vi "read pair information.vi"(8 "error in":errorcluster, 11 "UDP Broadcast Editor Node in":refnum<class "TEC editor node.lvclass">) -> (0 "error out":errorcluster, 2 "pair info":T1, 3 "UDP Broadcast Editor Node out":refnum<class "TEC editor node.lvclass">)   [LabVIEW 2013, in "TEC editor node.lvclass"]
uses:
  TEC editor node.lvclass
  pair information.ctl
  pair type.ctl
  TEC editor node.lvclass/TEC editor node.ctl
  <vilib>/NI/Tag Bus Module Framework/root configuration/TBM configuration.lvclass
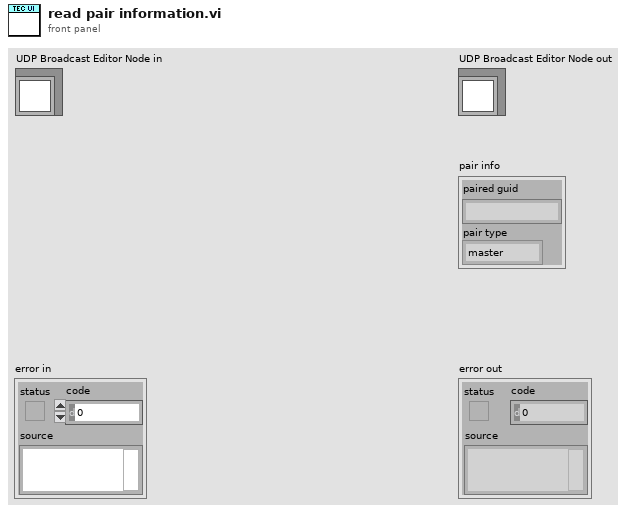
[diagram p1: front panel]
types:
  T1 = typedef "TEC editor node.lvclass/pair information.ctl" = cluster{"paired guid":string, "pair type":T2}
  T2 = typedef "TEC editor node.lvclass/pair type.ctl" = enum16{"master", "slave"}
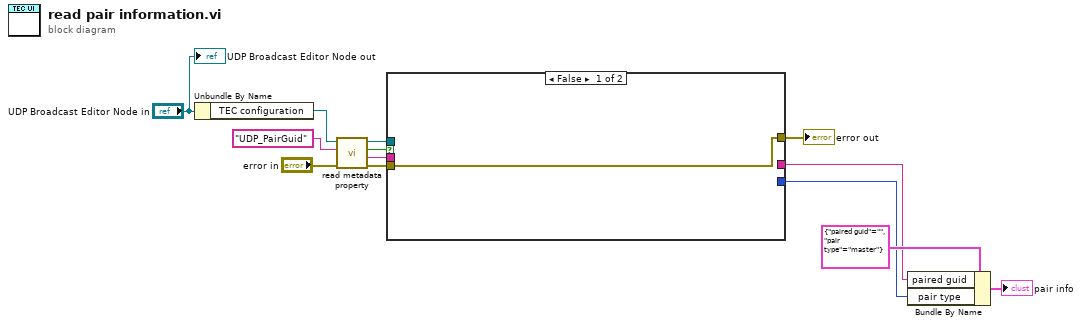
[diagram p0: block diagram]
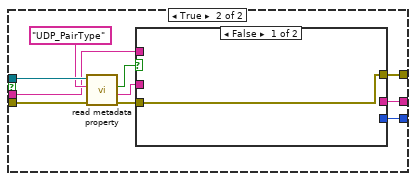
[diagram p2: hidden frame]
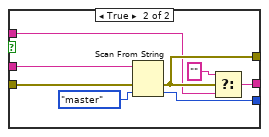
[diagram p3: hidden frame]
diagram:
  n1 = Unbundle By Name("UDP Broadcast Editor Node in") -> ("TEC configuration"=w11:refnum<class "TEC configuration.lvclass">)
  n2 = call <vilib>:"read metadata property.vi"("error in"="error in", "key"="UDP_PairGuid", "configuration in"=w11) -> ("error out"=w10:errorcluster, "value"=w3:string, "found"=w1:bool, "configuration out"=w12:refnum<class "TEC configuration.lvclass">)  [unwired: 5 in]
  n3 = case shown="False" w1 {
    tunnel: w12 -> [_ w24]
    tunnel: w10 -> [w14 w23]
    tunnel: [_ w18] -> w5
    tunnel: [w14 w17] -> w4
    tunnel: w3 -> [_ w16]
    tunnel: [_ w15] -> w2
    frame False {
    }
    frame True {
      n4 = call <vilib>:"read metadata property.vi"("error in"=w23, "key"="UDP_PairType", "configuration in"=w24) -> ("error out"=w19:errorcluster, "value"=w20:string, "found"=w21:bool)  [unwired: 5 in, 1 out]
      n5 = case shown="False" w21 {
        tunnel: w20 -> [_ w33]
        tunnel: w19 -> [w25 w32]
        tunnel: [_ w30] -> w18
        tunnel: [w25 w29] -> w17
        tunnel: w16 -> [_ w28]
        tunnel: [_ w26] -> w15
        frame False {
        }
        frame True {
          n6 = Scan From String(input string=w33, error in=w32, default 1=pair_type."master" ("pair type")) -> (error out=w29:errorcluster, output 1=w30:T2)  [unwired: 2 in, 2 out]
          n7 = Select(t="", s=w29, f=w28) -> (s? t:f=w26:string)
        }
      }
    }
  }
  "error out" <- w4
  n8 = Bundle By Name(cluster=T1 {"paired guid"="", "pair type"=enum."master"} ("pair info"), "paired guid"=w2, "pair type"=w5) -> (→"pair info":T1)
  "UDP Broadcast Editor Node out" <- "UDP Broadcast Editor Node in"
